vi "Get ID.vi"(11 "IConnection in":refnum<class "IConnection.lvclass">) -> (2 "ID":string)   [LabVIEW 2020, in "Connection Reference.lvlib" / "IConnection.lvclass"]
uses:
  <vilib>/gpm_packages/@cs/Network-interface/Source/Connection Reference/IConnection/IConnection.lvclass
  <vilib>/gpm_packages/@cs/Network-interface/Source/Connection Reference/IConnection/IConnection.lvclass/IConnection.ctl
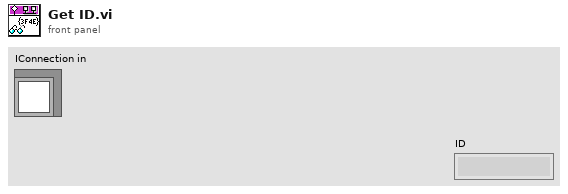
[diagram p1: front panel]
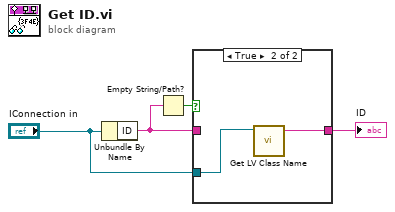
[diagram p0: block diagram]
diagram:
  n1 = Unbundle By Name("IConnection in") -> ("ID"=w2:string)
  n2 = Empty String/Path?(string/path=w2) -> (empty?=w3:bool)
  n3 = case shown="True" w3 {
    tunnel: "IConnection in" -> [_ w7]
    tunnel: w2 -> [w5 _]
    tunnel: [w5 w6] -> w1
    frame False {
    }
    frame True {
      n4 = call <vilib>:"Get LV Class Name.vi"("object"=w7) -> ("class name"=w6:string)  [unwired: 9 in, 1 out]
    }
  }
  "ID" <- w1
